vi "SwerveJoystickLogic.vi"(8 "Gyro":dbl, 9 "TankMode":bool, 10 "Joystick Axes":dbl[](array[numeric])) -> (2 "Speeds":dbl[](array[numeric]), 3 "Angles":dbl[](array[numeric]))   [LabVIEW 2019]
uses:
  Driver Globals.vi
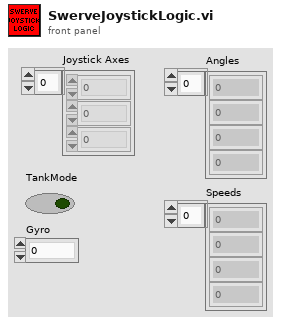
[diagram p1: front panel]
types:
  T1 = typedef "WPI_DriverStationRobotMode2.ctl" = enum16{"Autonomous Disabled", "Autonomous Enabled", "Teleop Disabled", "Teleop Enabled", "Disconnected", "Finish", "Test Disabled", "Test Enabled", "Emergency Stopped"}
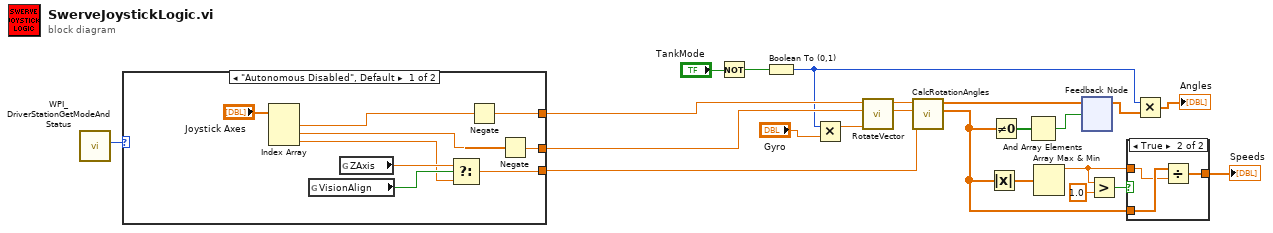
[diagram p0: block diagram]
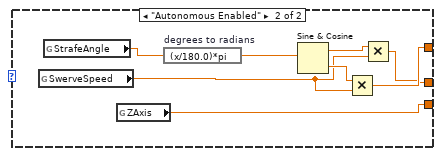
[diagram p2: hidden frame]
diagram:
  n1 = call <vilib>:"WPI_DriverStationGetModeAndStatus.vi"() -> ("Robot Mode"=w1:T1)  [unwired: 10 in, 1 out]
  n2 = case shown="\"Autonomous Disabled\", Default" w1 {
    tunnel: [w27 w33] -> w14
    tunnel: [w31 w32] -> w13
    tunnel: [w25 w39] -> w12
    frame "Autonomous Disabled", Default {
      n3 = Index Array(array="Joystick Axes") -> (element #1=w28:dbl, element #2=w30:dbl, element #3=w23:dbl)  [unwired: 3 in]
      n4 = global read "Driver Globals.vi" "VisionAlign"() -> (w26:bool)
      n5 = global read "Driver Globals.vi" "ZAxis"() -> (w24:dbl)
      n6 = Select(t=w24, s=w26, f=w23) -> (s? t:f=w25:dbl)
      n7 = Negate(x=w28) -> (-x=w27:dbl)
      n8 = Negate(x=w30) -> (-x=w31:dbl)
    }
    frame "Autonomous Enabled" {
      n9 = global read "Driver Globals.vi" "SwerveSpeed"() -> (w34:dbl)
      n10 = global read "Driver Globals.vi" "StrafeAngle"() -> (w38:dbl)
      n11 = global read "Driver Globals.vi" "ZAxis"() -> (w39:dbl)
      n12 = expression code="(x/180.0)*pi" "degrees to radians"(w38) -> (w37:dbl)
      n13 = Sine & Cosine(0:w37) -> (1:w36:dbl, 2:w35:dbl)
      n14 = Multiply(x=w35, y=w34) -> (x*y=w33:dbl)
      n15 = Multiply(x=w36, y=w34) -> (x*y=w32:dbl)
    }
  }
  n16 = Not(x="TankMode") -> (.not. x?=w7:bool)
  n17 = Boolean To (0,1)(Boolean=w7) -> (0, 1=w2:i16)
  n18 = Multiply(x=w2, y="Gyro") -> (x*y=w6:dbl)
  n19 = call "RotateVector.vi"("Angle"=w6, "Y"=w13, "X"=w14) -> ("Y'"=w9:dbl, "X'"=w10:dbl)  [unwired: 6 in]
  n20 = call "CalcRotationAngles.vi"("ZAxis"=w12, "YAxis"=w9, "XAxis"=w10) -> ("Speeds"=w18:dbl[], "Angles"=w17:dbl[])  [unwired: 7 in]
  n21 = Absolute Value(x=w18) -> (abs(x)=w19:dbl[])
  n22 = Not Equal To 0?(x=w18) -> (x != 0?=w11:bool[])
  n23 = And Array Elements(Boolean array=w11) -> (logical AND=w16:bool)
  n24 = Array Max & Min(array=w19) -> (max value=w20:dbl)  [unwired: 3 out]
  n25 = feedback #1() -> (w4:dbl[])  [unwired: 1 in]
  n26 = feedback-in #1(w17, w16) -> ()
  n27 = Greater?(x=w20, y=1.0) -> (0:w22:bool)
  n28 = case shown="True" w22 {
    tunnel: w18 -> [w40 w43]
    tunnel: w20 -> [_ w42]
    tunnel: [w40 w41] -> w15
    frame False {
    }
    frame True {
      n29 = Divide(x=w43, y=w42) -> (x/y=w41:dbl[])
    }
  }
  "Speeds" <- w15
  n30 = Multiply(x=w2, y=w4) -> (x*y=→"Angles":dbl[])
